vi "Check if Connection Allowed.vi"(8 "error in (no error)":errorcluster, 11 "TCP Slave in":refnum<class "TCP Slave.lvclass">) -> (0 "error out":errorcluster, 2 "Connection Allowed":bool, 3 "TCP Slave out":refnum<class "TCP Slave.lvclass">)   [LabVIEW 2021, in "TCP Slave.lvclass"]
doc: "Checks to see if a new connection is allowed."
uses:
  TCP Slave.lvclass
  TCP Slave.lvclass/TCP Slave.ctl
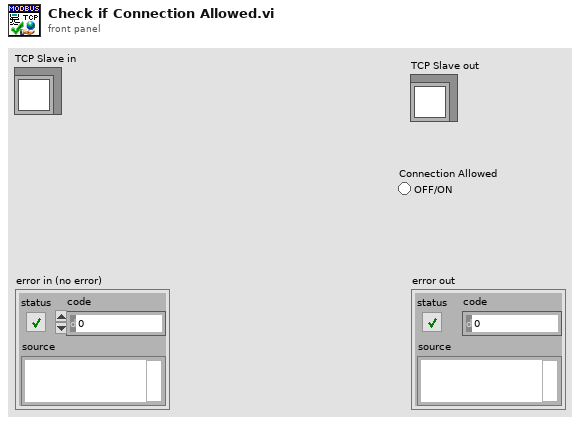
[diagram p1: front panel]
types:
  T1 = typedef "TCP Slave.lvclass/Connection Counter.ctl" = cluster{"Currently Connected":u32, "Connection Records":refnum<data-value>[]}
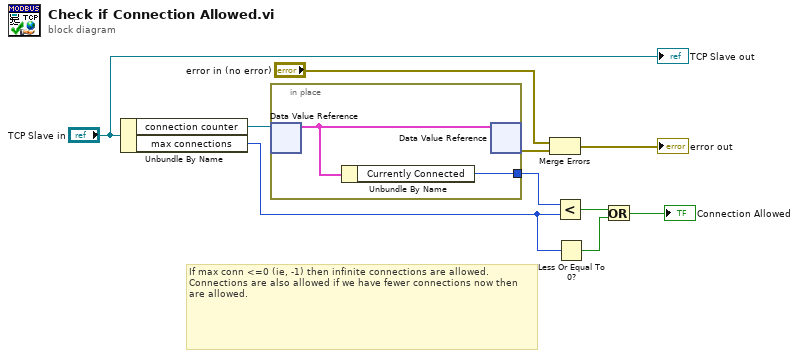
[diagram p0: block diagram]
diagram:
  # "If max conn <=0 (ie, -1) then infinite connections are allowed. Connections are also allowed if we have fewer connections now then are allowed."
  n1 = Unbundle By Name("TCP Slave in") -> ("connection counter"=w4:refnum<data-value>, "max connections"=w7:i32)
  n2 = in-place {
    in-place-border: [w11] -> w1
    n3 = in-place-dvr #1(w4) -> (w12:T1)  [unwired: 1 out]
    n4 = Unbundle By Name(w12) -> ("Currently Connected"=w11:u32)
    n5 = in-place-dvr #1(w12) -> (w5:errorcluster)  [unwired: 1 out]
  }
  n6 = Merge Errors("error in (no error)", w5) -> (→"error out":errorcluster)
  n7 = Less?(x=w1, y=w7) -> (x < y?=w2:bool)
  n8 = Less Or Equal To 0?(x=w7) -> (x <= 0?=w3:bool)
  n9 = Or(x=w2, y=w3) -> (x .or. y?=→"Connection Allowed":bool)
  "TCP Slave out" <- "TCP Slave in"
